vi "Get Waveform Attribute.vi"(8 "error in (no error)":errorcluster, 9 "Arb Name":string="EXP_RISE", 10 "Attribute (Average)":T1(ring), 11 "VISA resource name":refnum<visa-resource-name>) -> (0 "error out":errorcluster, 2 "Value":string, 3 "VISA resource name out":refnum<visa-resource-name>)   [LabVIEW 2017, in "Keithley 3390.lvlib"]
doc: "This VI retrieves the value of various attributes of a loaded arbitrary waveform."
uses:
  Keithley 3390.lvlib
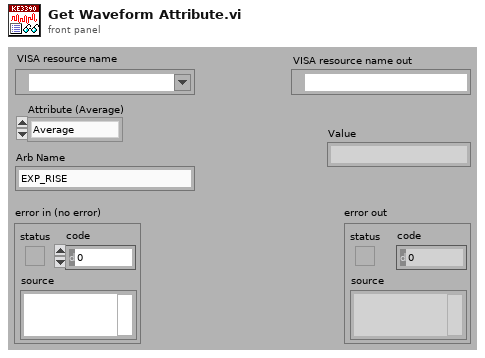
[diagram p1: front panel]
types:
  T1 = enum16{"Average", "Crest Factor", "Points", "Peak-To-Peak"}
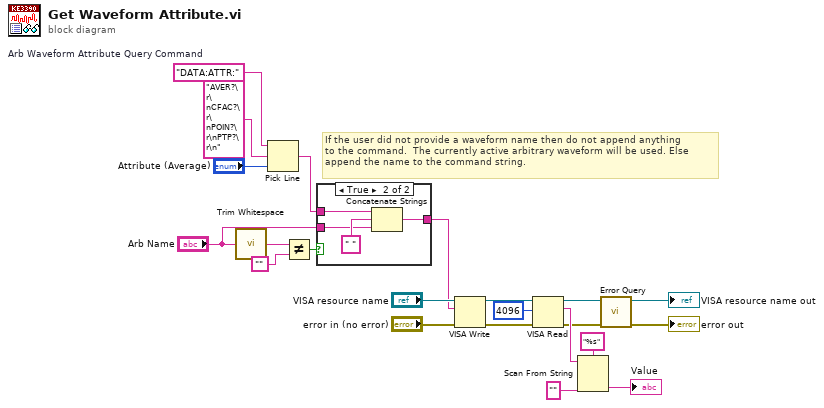
[diagram p0: block diagram]
diagram:
  w1 = "DATA:ATTR:"  # Arb Waveform Attribute Query Command
  # "If the user did not provide a waveform name then do not append anything\nto the command.  The currently active arbitrary waveform will be used. Else\nappend the name to the command string."
  n1 = call <vilib>:"Trim Whitespace.vi"("string"="Arb Name") -> ("trimmed string"=w5:string)  [unwired: 1 in]
  n2 = Pick Line(string ("")=w1, multi-line string="AVER?\r\nCFAC?\r\nPOIN?\r\nPTP?\r\n" ("options"), line index="Attribute (Average)") -> (output string=w19:string)
  n3 = Not Equal?(x=w5, y="") -> (x != y?=w3:bool)
  n4 = case shown="True" w3 {
    tunnel: w19 -> [w23 w27]
    tunnel: [w23 w26] -> w17
    tunnel: "Arb Name" -> [_ w24]
    frame False {
    }
    frame True {
      n5 = Concatenate Strings(w27, " " ("command"), w24) -> (w26:string)
    }
  }
  n6 = VISA Write(VISA resource name="VISA resource name", write buffer=w17, error in (no error)="error in (no error)") -> (VISA resource name out=w16:refnum<visa-resource-name>, error out=w15:errorcluster)  [unwired: 1 out]
  n7 = VISA Read(VISA resource name=w16, byte count=u32 4096, error in (no error)=w15) -> (VISA resource name out=w9:refnum<visa-resource-name>, read buffer=w13:string, error out=w8:errorcluster)  [unwired: 1 out]
  n8 = Scan From String(format string="%s", input string=w13, default 1="" ("default value 1")) -> (output 1=→"Value":string)  [unwired: 2 in, 3 out]
  n9 = call "Error Query.vi"("error in (no error)"=w8, "VISA resource name"=w9) -> ("error out"=→"error out":errorcluster, "VISA resource name out"=→"VISA resource name out":refnum<visa-resource-name>)  [unwired: 6 in, 2 out]
